vi "Package Name.vi"(8 "error in (no error)":errorcluster, 11 "Build Specification Name":string) -> (0 "error out":errorcluster, 3 "Package Name":string)   [LabVIEW 2016]
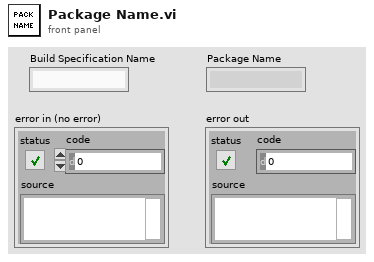
[diagram p1: front panel]
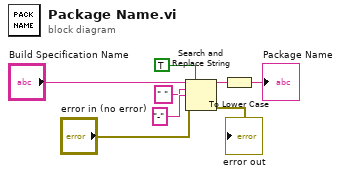
[diagram p0: block diagram]
diagram:
  n1 = Search and Replace String(replace all?=TRUE ("replace all? (F)"), input string="Build Specification Name", search string=" ", replace string="-" ("replace string (\"\")"), error in="error in (no error)") -> (result string=w4:string, error out=→"error out":errorcluster)  [unwired: 3 in, 2 out]
  n2 = To Lower Case(string=w4) -> (all lower case string=→"Package Name":string)
